vi "TS DotStar SPI V4.vi"() -> ()   [LabVIEW 2015]
doc: "ADXL362 SPI Accelerometer\n\nThis example shows how to use the Analog Devices ADXL362 Accelerometer sensor connected to SPI.\n\nThis example expects a USB cable connected from your development PC to the Type B USB Jack (next to the power input) on the roboRIO."
uses:
  <vilib>/Rock Robotics/SystemInterfaces/spilib/spi_bus.ctl
  <vilib>/Rock Robotics/WPI/SPI/WPI_SPIMode.ctl
panel:
  out "Aiming 2":bool
  out "Aiming":bool
  out "Intake":bool
  out "Shooter":bool
  in  "Slide":u8(slide) max=31 scale=0.0..31.0
  in  "Numeric 3":u8
  in  "Numeric 2":u8
  in  "Numeric":u8
  in  "Blue":bool
  in  "Red":bool
  in  "Green":bool
  in  "Number of Lights":u8
  in  "Number ON":u8
  in  "Chip Select Active High (F)":bool
  in  "Mode (3)":T1=enum."Mode 3 (Clk Idle High,Sample on Trailing)"
  in  "Clock Rate (Hz)":dbl=500000.0
  in  "error in":errorcluster
  in  "SPI Bus":T2=enum."SPI On-Board, CS1"
  out "error out":errorcluster
  in  "stop":bool
  # "Set these inputs before running."
  # "Number of Lights"
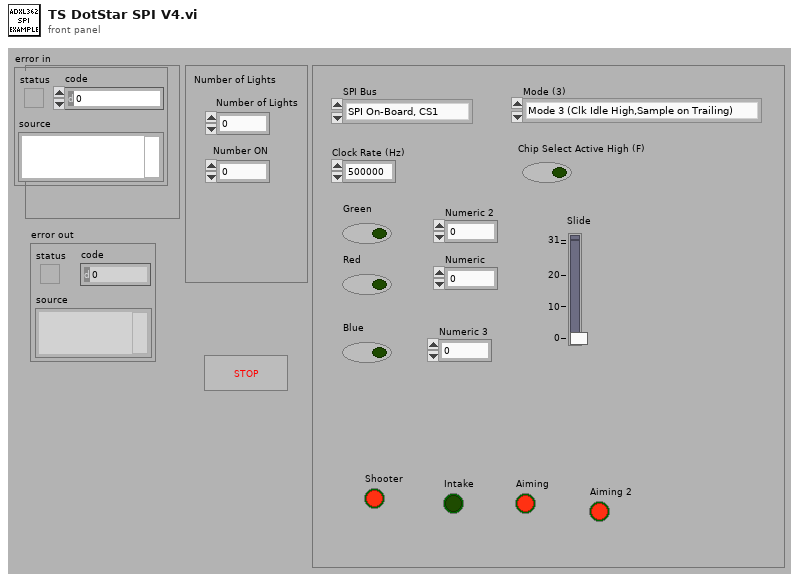
[diagram p1: front panel]
types:
  T1 = typedef "WPI_SPIMode.ctl" = enum16{"Mode 0 (Clk Idle Low,Sample on Leading)", "Mode 1 (Clk Idle Low,Sample on Trailing)", "Mode 2 (Clk Idle High,Sample on Leading)", "Mode 3 (Clk Idle High,Sample on Trailing)"}
  T2 = typedef "spi_bus.ctl" = enum16{"SPI On-Board, CS0", "SPI On-Board, CS1", "SPI On-Board, CS2", "SPI On-Board, CS3", "SPI MXP", "Invalid"}
  T3 = typedef "WPI_SPIDevRef.ctl" = cluster{"DevStatus":errorcluster, "Handle":i32, "SPI Bus":T2}
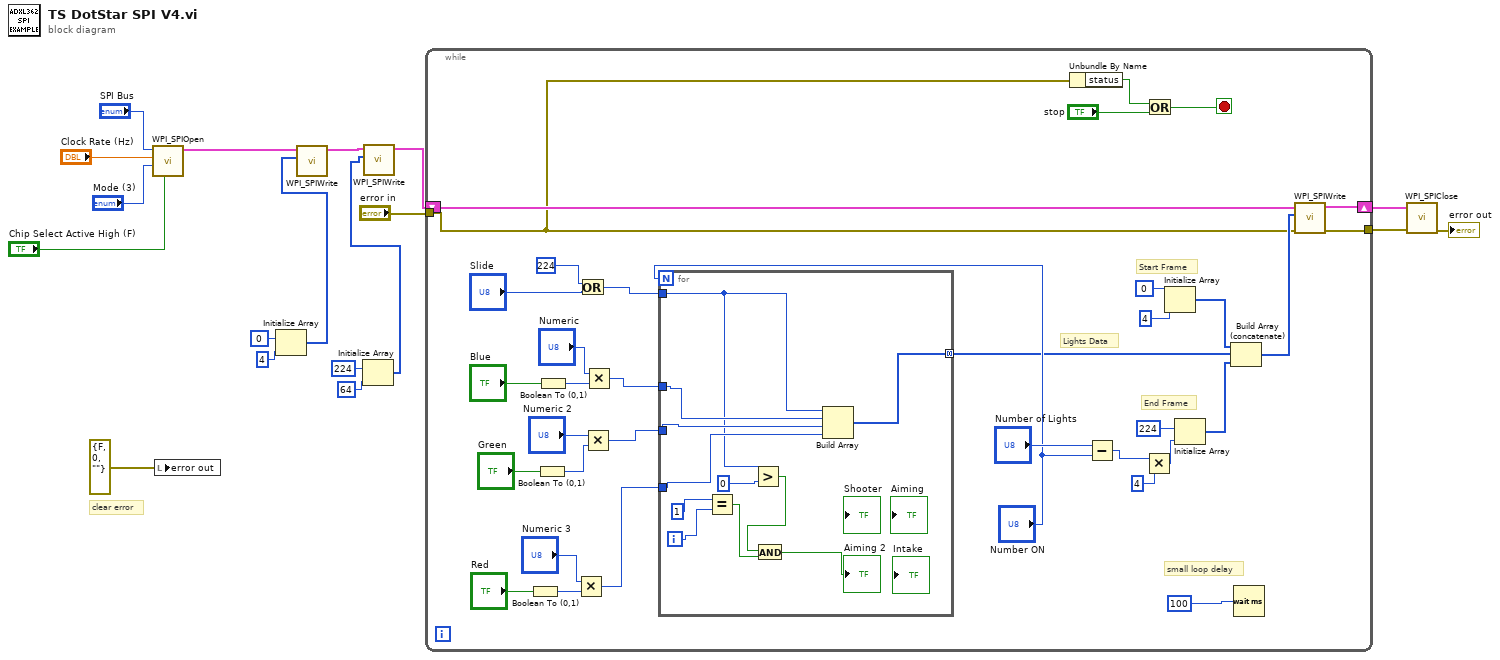
[diagram p0: block diagram]
diagram:
  # "clear error"
  n1 = call <vilib>:"WPI_SPIOpen.vi"("Chip Select Active High (F)"="Chip Select Active High (F)", "Mode (3)"="Mode (3)", "Clock Rate (Hz)"="Clock Rate (Hz)", "SPI Bus"="SPI Bus") -> ("SPIDevRef"=w8:T3)  [unwired: 6 in, 1 out]
  n2 = local write "error out"(errorcluster {"status"=FALSE, "code"=0, "source"=""} ("error out")) -> ()
  n3 = Initialize Array(u8 0 ("Data To Send"), u8 4 ("dimension size")) -> (w7:u8[])
  n4 = call <vilib>:"WPI_SPIWrite.vi"("Data To Send"=w7, "SPIDevRef"=w8) -> ("SPIDevRef"=w6:T3)  [unwired: 7 in, 2 out]
  n5 = Initialize Array(u8 224 ("Data To Send"), u8 64 ("dimension size")) -> (w2:u8[])
  n6 = call <vilib>:"WPI_SPIWrite.vi"("Data To Send"=w2, "SPIDevRef"=w6) -> ("SPIDevRef"=w5:T3)  [unwired: 7 in, 2 out]
  n7 = while {
    shift-right: [w48] -> w15
    shift-left: w5 -> [w26]
    tunnel: "error in" -> [w20]
    tunnel: [w47] -> w1
    stop <- w19 stop-if-true
    # "Lights Data"
    # "End Frame"
    # "Start Frame"
    # "small loop delay"
    n8 = Boolean To (0,1)(Boolean="Red") -> (0, 1=w40:i16)
    n9 = Boolean To (0,1)(Boolean="Green") -> (0, 1=w41:i16)
    n10 = Boolean To (0,1)(Boolean="Blue") -> (0, 1=w42:i16)
    n11 = Multiply(x="Numeric 3", y=w40) -> (x*y=w34:i16)
    n12 = Or(x=u8 224, y="Slide") -> (x .or. y?=w31:u8)
    n13 = Multiply(x="Numeric 2", y=w41) -> (x*y=w35:i16)
    n14 = Multiply(x="Numeric", y=w42) -> (x*y=w36:i16)
    n15 = for {
      N: "Number ON" -> [_]
      tunnel: w36 -> [w64]
      tunnel: w35 -> [w63]
      tunnel: w34 -> [w62]
      tunnel: w31 -> [w57]
      tunnel: [w61] -> w24 mode=concatenating
      i -> [w60]
      n16 = Equal?(x=u8 1 ("dimension size"), y=w60) -> (x = y?=w58:bool)
      n17 = Greater?(x=w57, y=u8 0 ("dimension size")) -> (0:w55:bool)
      n18 = And(x=w55, y=w58) -> (x .and. y?=→"Aiming 2":bool)
      n19 = Build Array(w57, w64, w63, w62) -> (w61:i16[])
    }
    n20 = Unbundle By Name(w20) -> ("status"=w21:bool)
    n21 = Subtract(x="Number of Lights", y="Number ON") -> (x-y=w27:u8)
    n22 = Multiply(x=w27, y=u8 4 ("dimension size")) -> (x*y=w30:u8)
    n23 = Or(x=w21, y="stop") -> (x .or. y?=w19:bool)
    n24 = Initialize Array(u8 0 ("Data To Send"), u8 4 ("dimension size")) -> (w25:u8[])
    n25 = Initialize Array(u8 224 ("Data To Send"), w30) -> (w23:u8[])
    n26 = Build Array (concatenate)(w25, w24, w23) -> (w22:i16[])
    n27 = Wait (ms)(milliseconds to wait=u32 100) -> ()  [unwired: 1 out]
    n28 = call <vilib>:"WPI_SPIWrite.vi"("error in (no error)"=w20, "Data To Send"=w22, "SPIDevRef"=w26) -> ("error out"=w47:errorcluster, "SPIDevRef"=w48:T3)  [unwired: 6 in, 1 out]
  }
  n29 = call <vilib>:"WPI_SPIClose.vi"("error in (no error)"=w1, "SPIDevRef"=w15) -> ("error out"=→"error out":errorcluster)  [unwired: 9 in]
